vi "Wavelength Meter.vi"(8 "error in (no error)":errorcluster, 11 "Wavelength Meter in":refnum<class "Wavelength Meter.lvclass">) -> (0 "error out":errorcluster, 3 "Wavelength Meter out":refnum<class "Wavelength Meter.lvclass">)   [LabVIEW 2009, in "Wavelength Meter.lvclass"]
uses:
  Wavelength Meter.lvclass
  <vilib>/Utility/error.llb/DialogType.ctl
  Utility Classes/Readable/Channel Units.ctl
  Utility Classes/Readable/Channel Names.ctl
  HighFinesse WS5/Variable Typedefs.llb/WLM control mode.ctl
  HighFinesse WS5/Variable Typedefs.llb/Exposure Mode.ctl
  Wavelength Meter.lvclass/Wavelength Meter.ctl
  Utility Classes/Readable/Readable.lvclass
  HighFinesse WS5/HighFinesse WS5.lvlib
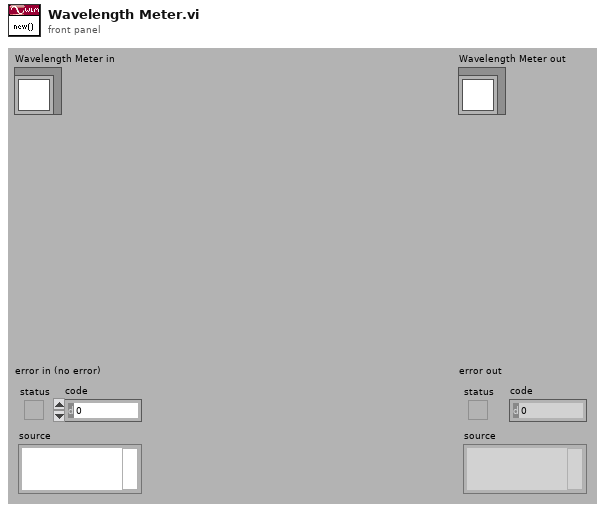
[diagram p1: front panel]
types:
  T1 = typedef "Readable.lvclass/Channel Units.ctl" = string[]
  T2 = typedef "Readable.lvclass/Channel Names.ctl" = string[]
  T3 = typedef "DialogType.ctl" = u16
  T4 = typedef "HighFinesse WS5.lvlib/WLM control mode.ctl" = i16
  T5 = typedef "HighFinesse WS5.lvlib/Exposure Mode.ctl" = enum16{"manual", "automatic"}
  T6 = enum16{"Measurement off", "Adjustment mode", "Measurement mode"}
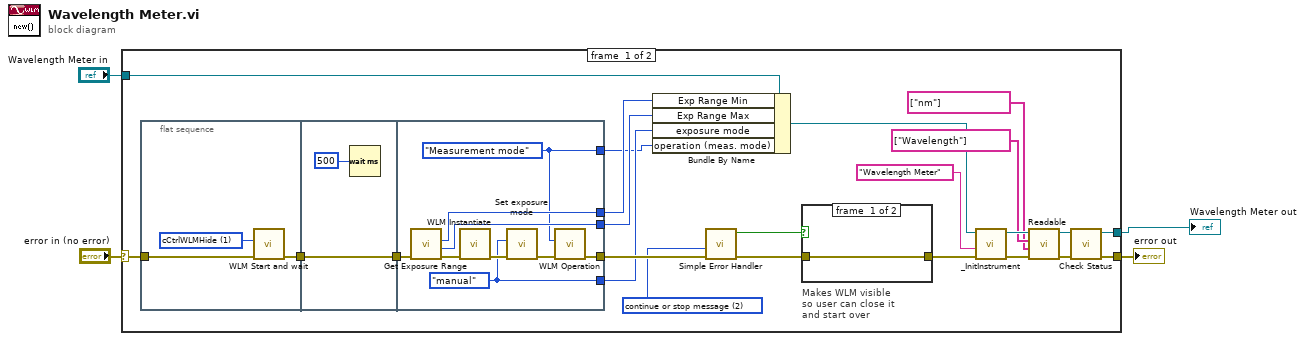
[diagram p0: block diagram]
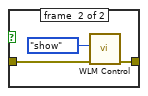
[diagram p2: hidden frame]
diagram:
  n1 = case shown="No Error" "error in (no error)" {
    selector: "error in (no error)" -> [w22 w47]
    tunnel: [w13 w47] -> w3
    tunnel: [w12 w46] -> w1
    tunnel: "Wavelength Meter in" -> [w19 w46]
    frame #0 {
      w10 = T3 2 items=["no dialog", "OK message", "continue or stop message", "OK message + warnings", "continue/stop + warnings"] ("type of dialog (OK msg:1)")
      n2 = flat-sequence {
        tunnel: w22 -> [w34]
        tunnel: [w33] -> w20
        tunnel: [w35] -> w21
        tunnel: w20 -> [w35]
        tunnel: [w43] -> w11
        tunnel: w21 -> [w42]
        tunnel: [w40] -> w18
        tunnel: [w39] -> w17
        tunnel: [w38] -> w9
        tunnel: [w37] -> w8
        frame #0 {
          w32 = T4 1 items=["cCtrlWLMShow", "cCtrlWLMHide", "cCtrlWLMExit"] ("WLM Control Mode Constants")
          n3 = call "WLM Start and wait.vi"("error in (no error)"=w34, "WLM Control Mode Constants"=w32) -> ("error out"=w33:errorcluster)  [unwired: 9 out]
        }
        frame #1 {
          n4 = Wait (ms)(milliseconds to wait=u32 500) -> ()  [unwired: 1 out]
        }
        frame #2 {
          w38 = Exposure_Mode."manual" ("exposure mode")
          w37 = T6."Measurement mode" ("operation (meas. mode)")
          n5 = call "Get Exposure Range.vi"("error in (no error)"=w42) -> ("error out"=w41:errorcluster, "Exp Range Max"=w39:u32, "Exp Range Min"=w40:u32)  [unwired: 8 in]
          n6 = call "WLM Instantiate.vi"("error in (no error)"=w41) -> ("error out"=w45:errorcluster)  [unwired: 9 in, 1 out]
          n7 = call "Set exposure mode.vi"("error in (no error)"=w45, "exposure mode"=w38) -> ("error out"=w44:errorcluster)  [unwired: 9 out]
          n8 = call "WLM Operation.vi"("error in (no error)"=w44, "operation (meas. mode)"=w37) -> ("error out"=w43:errorcluster)  [unwired: 9 out]
        }
      }
      n9 = Bundle By Name(cluster=w19, "Exp Range Min"=w18, "Exp Range Max"=w17, "exposure mode"=w9, "operation (meas. mode)"=w8) -> (w16:refnum<class "Wavelength Meter.lvclass">)
      n10 = call <vilib>:"Simple Error Handler.vi"("type of dialog (OK msg:1)"=w10, "error in (no error)"=w11) -> ("error?"=w7:bool, "error out"=w6:errorcluster)  [unwired: 3 in, 3 out]
      n11 = case "Makes WLM visible\nso user can close it\nand start over" shown="True" w7 {
        tunnel: w6 -> [w28 w30]
        tunnel: [w28 w29] -> w5
        frame #0 {
        }
        frame #1 {
          n12 = call "WLM Control.vi"("error in (no error)"=w30, "command"=enum16{"show", "hide", "exit"}."show") -> ("error out"=w29:errorcluster)  [unwired: 9 out]
        }
      }
      n13 = call-dynamic "_InitInstrument.vi"("error in (no error)"=w5, "Name"="Wavelength Meter", "Instrument in"=w16) -> ("error out"=w26:errorcluster, "Instrument out"=w25:refnum<class "Wavelength Meter.lvclass">)  [unwired: 3 in, 4 out]
      n14 = call "Readable.vi"("error in (no error)"=w26, "Channel Units"=T1 ["nm"], "Channel Names"=T2 ["Wavelength"], "Readable in"=w25) -> ("error out"=w14:errorcluster, "Readable out"=w15:refnum<class "Wavelength Meter.lvclass">)  [unwired: 6 in]
      n15 = call-dynamic "Check Status.vi"("error in (no error)"=w14, "Wavelength Meter in"=w15) -> ("error out"=w13:errorcluster, "Wavelength Meter out"=w12:refnum<class "Wavelength Meter.lvclass">)  [unwired: 6 in, 2 out]
    }
    frame #1 {
    }
  }
  "error out" <- w3
  "Wavelength Meter out" <- w1
